vi "calculate_trnsformator_coef.vi"(8 "error in (no error)":errorcluster, 10 "voltage":dbl, 11 "UI in":T1) -> (0 "error out":errorcluster, 2 "koef":dbl, 3 "UI out 2":T1)   [LabVIEW 2017]
uses:
  ui.ctl
  classes/dc_power_supply/DC_power_supply.lvclass
  classes/report/Report.lvclass
  ui_buttons.ctl
  types/boc_type.ctl
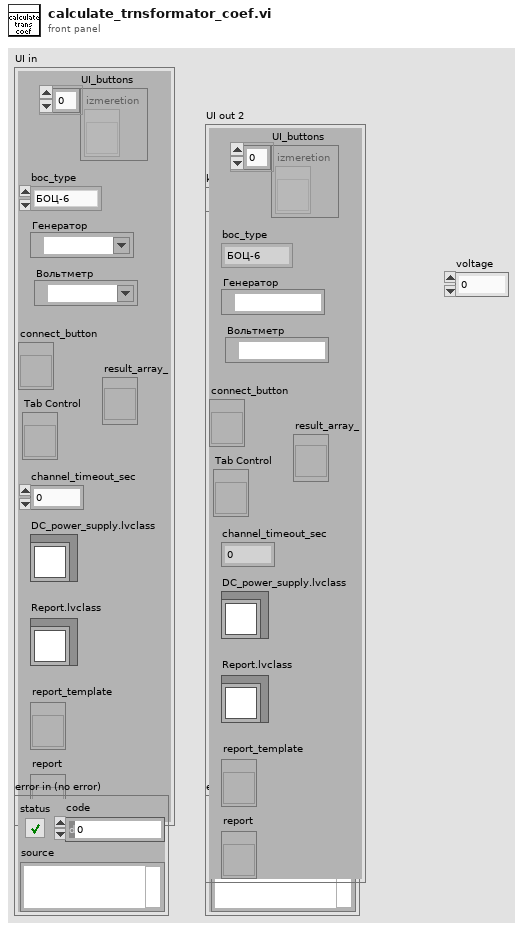
[diagram p1: front panel]
types:
  T1 = typedef "ui.ctl" = cluster{"UI_buttons":T2, "Tab Control":refnum<vi>, "connect_button":refnum<vi>, "generator":refnum<visa-resource-name>, "voltmetr":refnum<visa-resource-name>, "channel_timeout_sec":dbl, "boc_type":T3, "result_array_":refnum<vi>, "DC_power_supply.lvclass":refnum<class "DC_power_supply.lvclass">, "Report.lvclass":refnum<class "Report.lvclass">, "report_template":refnum<vi>, "report":refnum<vi>}
  T2 = typedef "ui_buttons.ctl" = refnum<vi>[]
  T3 = typedef "boc_type.ctl" = enum16{"БОЦ-6", "БОЦ-12"}
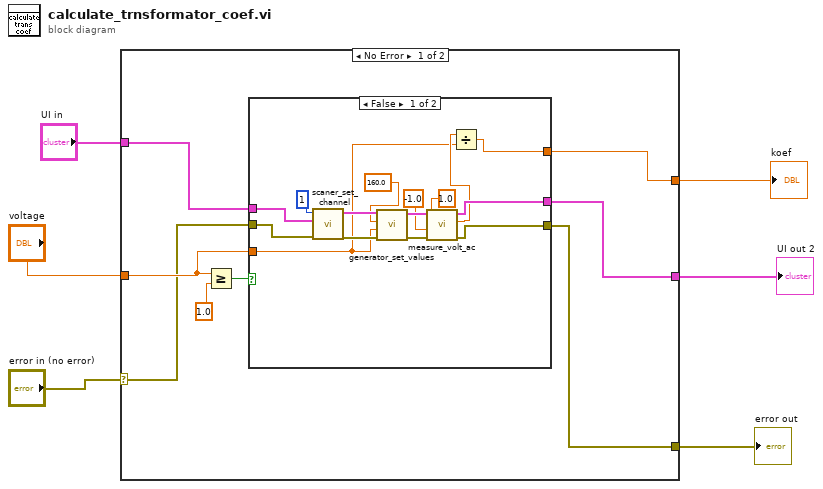
[diagram p0: block diagram]
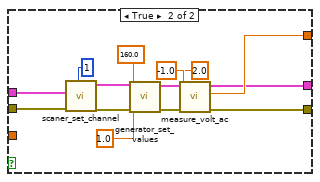
[diagram p2: hidden frame]
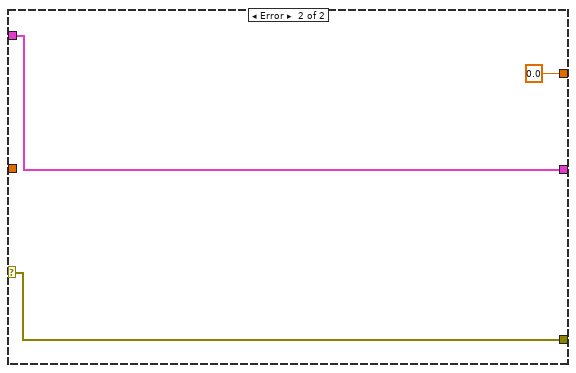
[diagram p3: hidden frame]
diagram:
  n1 = case shown="No Error" "error in (no error)" {
    selector: "error in (no error)" -> [w7 w45]
    tunnel: "UI in" -> [w14 w46]
    tunnel: [w13 0.0 ("Measurement")] -> w5
    tunnel: [w12 w45] -> w4
    tunnel: [w11 w46] -> w3
    tunnel: "voltage" -> [w8 _]
    frame No Error {
      n2 = Greater Or Equal?(x=w8, y=1.0) -> (x >= y?=w9:bool)
      n3 = case shown="False" w9 {
        tunnel: w14 -> [w21 w41]
        tunnel: w7 -> [w20 w40]
        tunnel: [w15 w38] -> w13
        tunnel: [w18 w32] -> w12
        tunnel: [w19 w31] -> w11
        tunnel: w8 -> [w16 _]
        frame False {
          n4 = call "scaner_set_channel.vi"("error in (no error)"=w20, "UI in"=w21, "Numeric"=1) -> ("error out"=w27:errorcluster, "UI_out"=w26:T1)  [unwired: 7 in]
          n5 = call "generator_set_values.vi"("error in (no error)"=w27, "Amplitude (1.0 Vpp)"=w16, "freq_value"=160.0, "UI in"=w26) -> ("error out"=w28:errorcluster, "UI_out"=w29:T1)  [unwired: 6 in]
          n6 = call "measure_volt_ac.vi"("error in (no error)"=w28, "Resolution"=-1.0, "Range"=1.0, "UI in in"=w29) -> ("error out"=w18:errorcluster, "Measurement"=w17:dbl, "UI out"=w19:T1)  [unwired: 5 in]
          n7 = Divide(x=w17, y=w16) -> (x/y=w15:dbl)
        }
        frame True {
          n8 = call "scaner_set_channel.vi"("error in (no error)"=w40, "UI in"=w41, "Numeric"=1) -> ("error out"=w39:errorcluster, "UI_out"=w42:T1)  [unwired: 7 in]
          n9 = call "generator_set_values.vi"("error in (no error)"=w39, "Amplitude (1.0 Vpp)"=1.0, "freq_value"=160.0, "UI in"=w42) -> ("error out"=w33:errorcluster, "UI_out"=w30:T1)  [unwired: 6 in]
          n10 = call "measure_volt_ac.vi"("error in (no error)"=w33, "Resolution"=-1.0, "Range"=2.0, "UI in in"=w30) -> ("error out"=w32:errorcluster, "Measurement"=w38:dbl, "UI out"=w31:T1)  [unwired: 5 in]
        }
      }
    }
    frame Error {
    }
  }
  "koef" <- w5
  "error out" <- w4
  "UI out 2" <- w3
